vi "CanBurglarAuto.vi"(8 "error in":errorcluster) -> (0 "error out":errorcluster)   [LabVIEW 2014]
uses:
  Utilities/CanGrabberSetpoint.vi
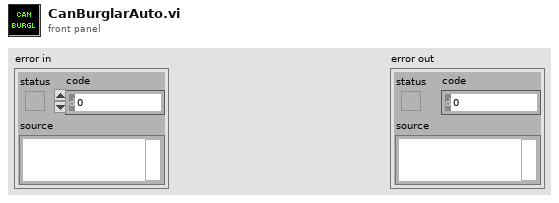
[diagram p1: front panel]
types:
  T1 = typedef "WPI_MotorControlDeviceRef.ctl" = cluster{"DeviceStatus":errorcluster, "Type":T2, "PWM":cluster{"Controller":T3, "PWM Channel":T4, "DeadBand":T5}, "CAN":cluster{"Device Number":u8, "Control Mode":T6, "Semaphore":T7, "Max Vout":dbl, "TalonSRX Control Mode":T8}, "Invert":bool, "TransformRef":T9, "InvTransformRef":T9}
  T2 = typedef "WPI_MotorControlType.ctl" = enum16{"PWM", "CAN", "CANTalonSRX"}
  T3 = typedef "FPGA_TypedefDigitalModule.ctl" = enum16{"Controller 1"}
  T4 = typedef "FPGA_DIOPWMChannel.ctl" = enum8{"PWM 0", "PWM 1", "PWM 2", "PWM 3", "PWM 4", "PWM 5", "PWM 6", "PWM 7", "PWM 8", "PWM 9", "PWM MXP 0", "PWM MXP 1", "PWM MXP 2", "PWM MXP 3", "PWM MXP 4", "PWM MXP 5", "PWM MXP 6", "PWM MXP 7", "PWM MXP 8", "PWM MXP 9", "Invalid"}
  T5 = typedef "WPI_PWMDeadband.ctl" = cluster{"Name":string, "maxPositivePwm":i32, "minPositivePwm":i32, "centerPwm":i32, "maxNegativePwm":i32, "minNegativePwm":i32, "angularRange":u16}
  T6 = typedef "WPI_CANJaguar_ControlMode.ctl" = enum8{"Percent VBus", "Current", "Speed", "Position", "Voltage"}
  T7 = typedef "Semaphore RefNum" = refnum<k1>
  T8 = typedef "WPI_CANTalonSRX_APIControlMode.ctl" = enum8{"Percent VBus", "Speed", "Position", "Slave", "Unchanged / Invalid"}
  T9 = typedef "WPI_PWMTransform_ConPane.ctl" = refnum<vi>
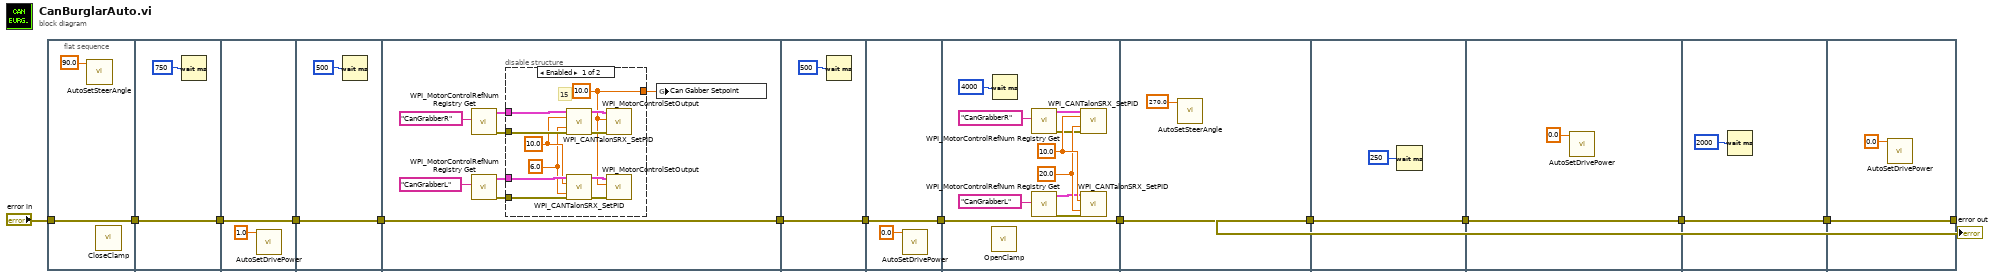
[diagram p0: block diagram]
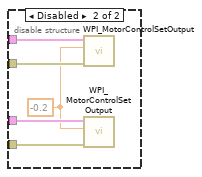
[diagram p2: hidden frame]
diagram:
  n1 = flat-sequence {
    tunnel: "error in" -> [w15]
    tunnel: [w15] -> w11
    tunnel: [w17] -> w12
    tunnel: w11 -> [w17]
    tunnel: [w20] -> w8
    tunnel: w12 -> [w20]
    tunnel: w8 -> [w22]
    tunnel: [w22] -> w7
    tunnel: w7 -> [w30]
    tunnel: [w30] -> w6
    tunnel: [w47] -> w13
    tunnel: w6 -> [w47]
    tunnel: w13 -> [w49]
    tunnel: [w49] -> w9
    tunnel: w9 -> [w60]
    tunnel: [w60] -> w5
    tunnel: w5 -> [w62]
    tunnel: [w62] -> w4
    tunnel: w4 -> [w64]
    tunnel: [w64] -> w3
    tunnel: w3 -> [w66]
    tunnel: [w66] -> w2
    tunnel: w2 -> [w68]
    tunnel: [w68] -> w1
    tunnel: [w70] -> w10
    tunnel: w1 -> [w70]
    frame #0 {
      n2 = call "AutoSetSteerAngle.vi"("Angle"=90.0) -> ()  [unwired: 11 in]
      n3 = call "CloseClamp.vi"() -> ()  [unwired: 12 in]
    }
    frame #1 {
      n4 = Wait (ms)(milliseconds to wait=u32 750) -> ()  [unwired: 1 out]
    }
    frame #2 {
      n5 = call "AutoSetDrivePower.vi"("Power"=1.0) -> ()  [unwired: 11 in]
    }
    frame #3 {
      n6 = Wait (ms)(milliseconds to wait=u32 500) -> ()  [unwired: 1 out]
    }
    frame #4 {
      n7 = call <vilib>:"WPI_MotorControlRefNum Registry Get.vi"("refnum name"="CanGrabberR") -> ("error out"=w24:errorcluster, "MotorControlDevRef"=w25:T1)  [unwired: 9 in]
      n8 = call <vilib>:"WPI_MotorControlRefNum Registry Get.vi"("refnum name"="CanGrabberL") -> ("error out"=w27:errorcluster, "MotorControlDevRef"=w28:T1)  [unwired: 9 in]
      n9 = disable-structure shown="Enabled" {
        disable-tunnel: w28 -> [w39 w44]
        disable-tunnel: w27 -> [w38 w43]
        disable-tunnel: w25 -> [w35 w46]
        disable-tunnel: w24 -> [w34 w45]
        disable-tunnel: [w31 _] -> w23
        frame Enabled {
          w32 = 6.0 ("D")
          w33 = 10.0 ("P")
          w31 = 10.0 ("Output")
          # "15"
          n10 = call <vilib>:"WPI_CANTalonSRX_SetPID.vi"("CAN Talon SRX Ref"=w35, "P"=w33, "D"=w32, "error in (no error)"=w34) -> ("CAN Talon SRX Ref Out"=w37:T1, "error out"=w36:errorcluster)  [unwired: 10 in]
          n11 = call <vilib>:"WPI_CANTalonSRX_SetPID.vi"("CAN Talon SRX Ref"=w39, "P"=w33, "D"=w32, "error in (no error)"=w38) -> ("CAN Talon SRX Ref Out"=w41:T1, "error out"=w40:errorcluster)  [unwired: 10 in]
          n12 = call <vilib>:"WPI_MotorControlSetOutput.vi"("error in (no error)"=w36, "Output"=w31, "MotorControlDevRef"=w37) -> ()  [unwired: 6 in, 3 out]
          n13 = call <vilib>:"WPI_MotorControlSetOutput.vi"("error in (no error)"=w40, "Output"=w31, "MotorControlDevRef"=w41) -> ()  [unwired: 6 in, 3 out]
        }
        frame Disabled {
          w42 = -0.2 ("Output")
          n14 = call <vilib>:"WPI_MotorControlSetOutput.vi"("error in (no error)"=w45, "Output"=w42, "MotorControlDevRef"=w46) -> ()  [unwired: 6 in, 3 out]
          n15 = call <vilib>:"WPI_MotorControlSetOutput.vi"("error in (no error)"=w43, "Output"=w42, "MotorControlDevRef"=w44) -> ()  [unwired: 6 in, 3 out]
        }
      }
      n16 = global write "CanGrabberSetpoint.vi" "Can Gabber Setpoint"(w23) -> ()
    }
    frame #5 {
      n17 = Wait (ms)(milliseconds to wait=u32 500) -> ()  [unwired: 1 out]
    }
    frame #6 {
      n18 = call "AutoSetDrivePower.vi"("Power"=0.0) -> ()  [unwired: 11 in]
    }
    frame #7 {
      w55 = 20.0 ("D")
      w56 = 10.0 ("P")
      n19 = call "OpenClamp.vi"() -> ()  [unwired: 12 in]
      n20 = Wait (ms)(milliseconds to wait=u32 4000) -> ()  [unwired: 1 out]
      n21 = call <vilib>:"WPI_MotorControlRefNum Registry Get.vi"("refnum name"="CanGrabberR") -> ("error out"=w53:errorcluster, "MotorControlDevRef"=w54:T1)  [unwired: 9 in]
      n22 = call <vilib>:"WPI_MotorControlRefNum Registry Get.vi"("refnum name"="CanGrabberL") -> ("error out"=w51:errorcluster, "MotorControlDevRef"=w52:T1)  [unwired: 9 in]
      n23 = call <vilib>:"WPI_CANTalonSRX_SetPID.vi"("CAN Talon SRX Ref"=w54, "P"=w56, "D"=w55, "error in (no error)"=w53) -> ()  [unwired: 10 in, 2 out]
      n24 = call <vilib>:"WPI_CANTalonSRX_SetPID.vi"("CAN Talon SRX Ref"=w52, "P"=w56, "D"=w55, "error in (no error)"=w51) -> ()  [unwired: 10 in, 2 out]
    }
    frame #8 {
      n25 = call "AutoSetSteerAngle.vi"("Angle"=270.0) -> ()  [unwired: 11 in]
    }
    frame #9 {
      n26 = Wait (ms)(milliseconds to wait=u32 250) -> ()  [unwired: 1 out]
    }
    frame #10 {
      n27 = call "AutoSetDrivePower.vi"("Power"=0.0) -> ()  [unwired: 11 in]
    }
    frame #11 {
      n28 = Wait (ms)(milliseconds to wait=u32 2000) -> ()  [unwired: 1 out]
    }
    frame #12 {
      n29 = call "AutoSetDrivePower.vi"("Power"=0.0) -> ()  [unwired: 11 in]
    }
  }
  "error out" <- w10
